vi "WT1800 Get Measurement.vi"(0 "VISA resource name":refnum<visa-resource-name>, 5 "Measure Item (1: Plural)":i32(ring)=1 items=["One", "Plural"], 7 "Number of Item (15)":i32=15 min=1 max=255, 9 "Timeout (10000 ms)":i32=10000 min=1, 11 "error in (no error)":errorcluster) -> (4 "VISA resource name out":refnum<visa-resource-name>, 6 "Function":string[](array[string]), 8 "Measurement":dbl[](array[numeric]), 15 "error out":errorcluster)   [LabVIEW 2021]
uses:
  <instrlib>/Yokogawa WT1800 Series/Yokogawa WT1800 Series.lvlib
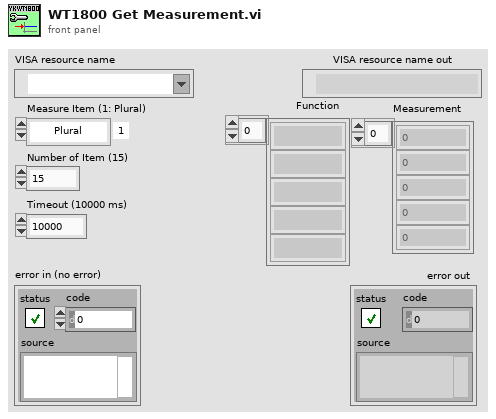
[diagram p1: front panel]
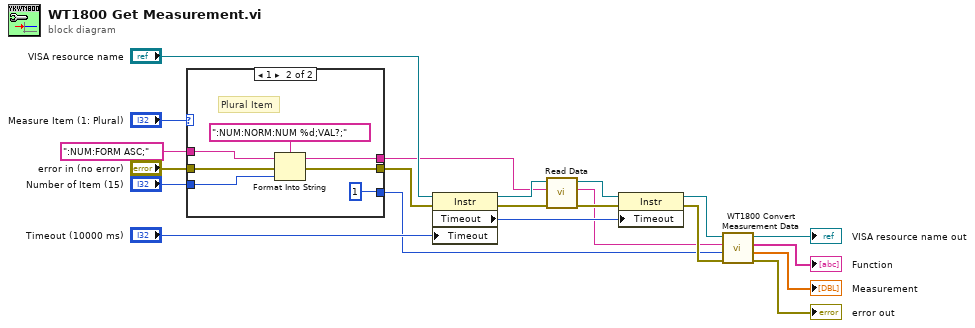
[diagram p0: block diagram]
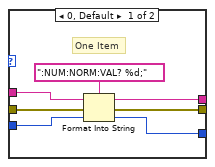
[diagram p2: hidden frame]
diagram:
  n1 = case shown="1" "Measure Item (1: Plural)" {
    tunnel: ":NUM:FORM ASC;" ("形式文字列") -> [w26 w33]
    tunnel: "Number of Item (15)" -> [w22 w32]
    tunnel: "error in (no error)" -> [w25 w31]
    tunnel: [w24 w30] -> w6
    tunnel: [w23 w29] -> w16
    tunnel: [w22 1] -> w11
    frame 0, Default {
      # "One Item"
      n2 = Format Into String(format string=":NUM:NORM:VAL? %d;" ("形式文字列"), initial string=w26, error in=w25, w22) -> (resulting string=w24:string, error out=w23:errorcluster)
    }
    frame 1 {
      # "Plural Item"
      n3 = Format Into String(format string=":NUM:NORM:NUM %d;VAL?;" ("形式文字列"), initial string=w33, error in=w31, w32) -> (resulting string=w30:string, error out=w29:errorcluster)
    }
  }
  n4 = property on="プロパティノード" class="Instr"(reference="VISA resource name", error in=w16, "Timeout"="Timeout (10000 ms)") -> (reference out=w7:refnum<visa-resource-name>, error out=w5:errorcluster, "Timeout"=w15:u32)
  n5 = call <instrlib>:"Read Data.vi"("error in (no error)"=w5, "Send Command (Empty)"=w6, "VISA resource name"=w7) -> ("error out"=w3:errorcluster, "Read Data"=w2:string, "VISA resource name out"=w4:refnum<visa-resource-name>)  [unwired: 5 in, 1 out]
  n6 = property on="プロパティノード" class="Instr"(reference=w4, error in=w3, "Timeout"=w15) -> (reference out=w13:refnum<visa-resource-name>, error out=w12:errorcluster)
  n7 = call "WT1800 Convert Measurement Data.vi"("error in (no error)"=w12, "Item Number Offset (1)"=w11, "Measurement Data (Empty)"=w2, "VISA resource name"=w13) -> ("error out"=→"error out":errorcluster, "Measurement"=→"Measurement":dbl[], "Function"=→"Function":string[], "VISA resource name out"=→"VISA resource name out":refnum<visa-resource-name>)  [unwired: 4 in]
